vi "SO55 Ion Source Main.vi"() -> ()   [LabVIEW 2012]
panel:
  out "AnodeCurrentInd":dbl format="%#.3g"
  out "Anode Current":dbl(knob) scale=0.0..10.0
  out "GasInd":dbl format="%#.3g"
  out "Gasmeter":dbl(knob) scale=0.0..40.0
  in  "Gas":dbl(knob) min=0.0 max=40.0 step=0.1 scale=0.0..40.0
  in  "ExitBtn":bool
  in  "SetBtn":bool
  out "AnodeInd":dbl format="%#.3g"
  out "Anodemeter":dbl(knob) scale=0.0..250.0 scale format="%-#3.3p"
  in  "Anode":dbl(knob) min=0.0 max=250.0 step=1.0 scale=0.0..250.0
  out "OvenInd":dbl format="%#.3g"
  out "MagInd":dbl format="%#.3g"
  out "FilInd":dbl format="%#.3g"
  out "Ovenmeter":dbl(knob) scale=0.0..40.0
  out "Magmeter":dbl(knob) scale=0.0..40.0
  out "Filmeter":dbl(knob) scale=0.0..40.0 scale format="%-#3.3p"
  in  "Oven":dbl(knob) min=0.0 max=40.0 step=0.1 scale=0.0..40.0
  in  "Mag":dbl(knob) min=0.0 max=30.0 step=0.1 scale=0.0..40.0
  in  "Fil":dbl(knob) min=0.0 max=40.0 step=0.1 scale=0.0..40.0
  # "Magnet"
  # "Oven"
  # "Gas"
  # "Anode"
  # "Filament"
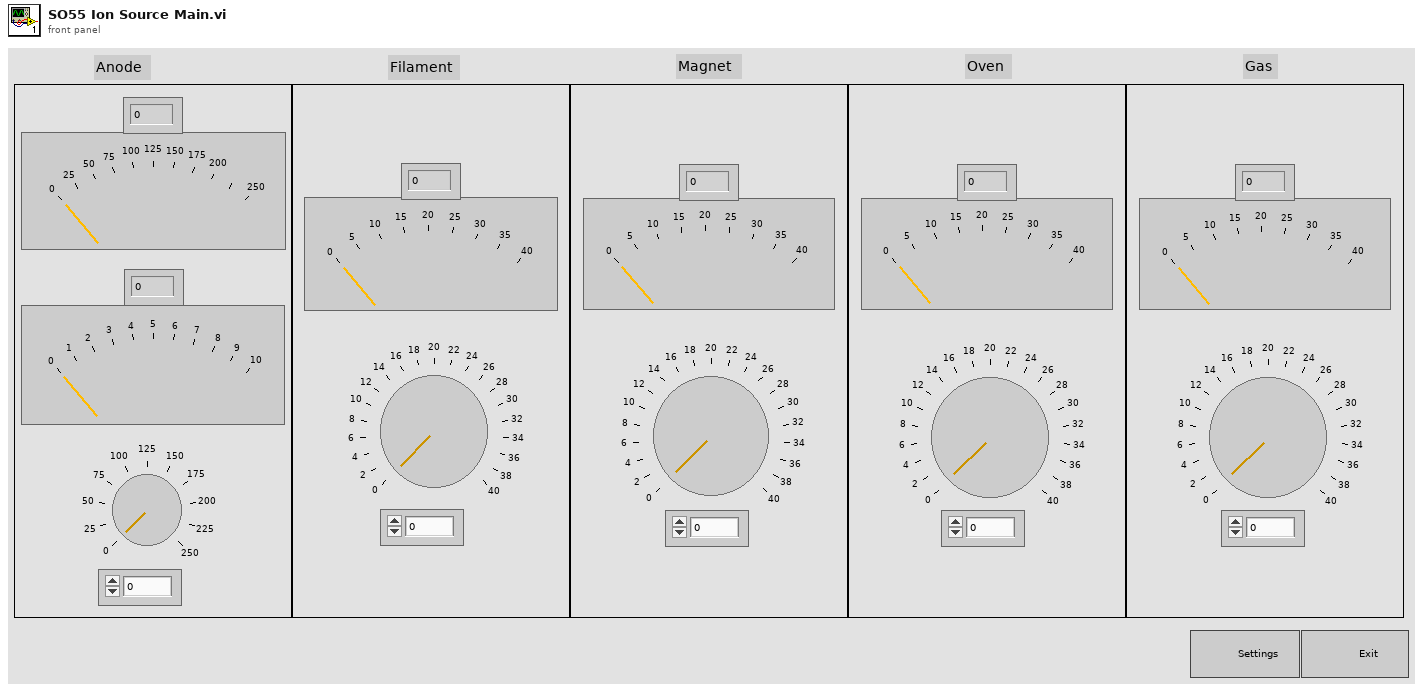
[diagram p1: front panel]
types:
  T1 = cluster{"Input":cluster{"Anode Input Channel":tag, "Filament Input Channel":tag, "Magnet Input Channel":tag, "Oven Input Channel":tag, "Gas Input Channel":tag, "Input Rate":dbl, "Anode Current Input Channel":tag}, "Output":cluster{"Anode":cluster{"Anode Output Channel":tag, "Anode Step":dbl}, "Filament":cluster{"Filament Output Channel":tag, "Filament Step":dbl}, "Magnet":cluster{"Magnet Output Channel":tag, "Magnet Step":dbl}, "Oven":cluster{"Oven Output Channel":tag, "Oven Step":dbl}, "Gas":cluster{"Gas Output Channel":tag, "Gas Step":dbl}, "Output Rate":dbl}}
  T2 = cluster{"Anode":cluster{"Anode Output Channel":tag, "Anode Step":dbl}, "Filament":cluster{"Filament Output Channel":tag, "Filament Step":dbl}, "Magnet":cluster{"Magnet Output Channel":tag, "Magnet Step":dbl}, "Oven":cluster{"Oven Output Channel":tag, "Oven Step":dbl}, "Gas":cluster{"Gas Output Channel":tag, "Gas Step":dbl}, "Output Rate":dbl}
  T3 = cluster{"Anode Input Channel":tag, "Filament Input Channel":tag, "Magnet Input Channel":tag, "Oven Input Channel":tag, "Gas Input Channel":tag, "Input Rate":dbl, "Anode Current Input Channel":tag}
  T4 = enum8{"Enabled", "Disabled", "Disabled and Grayed Out"}
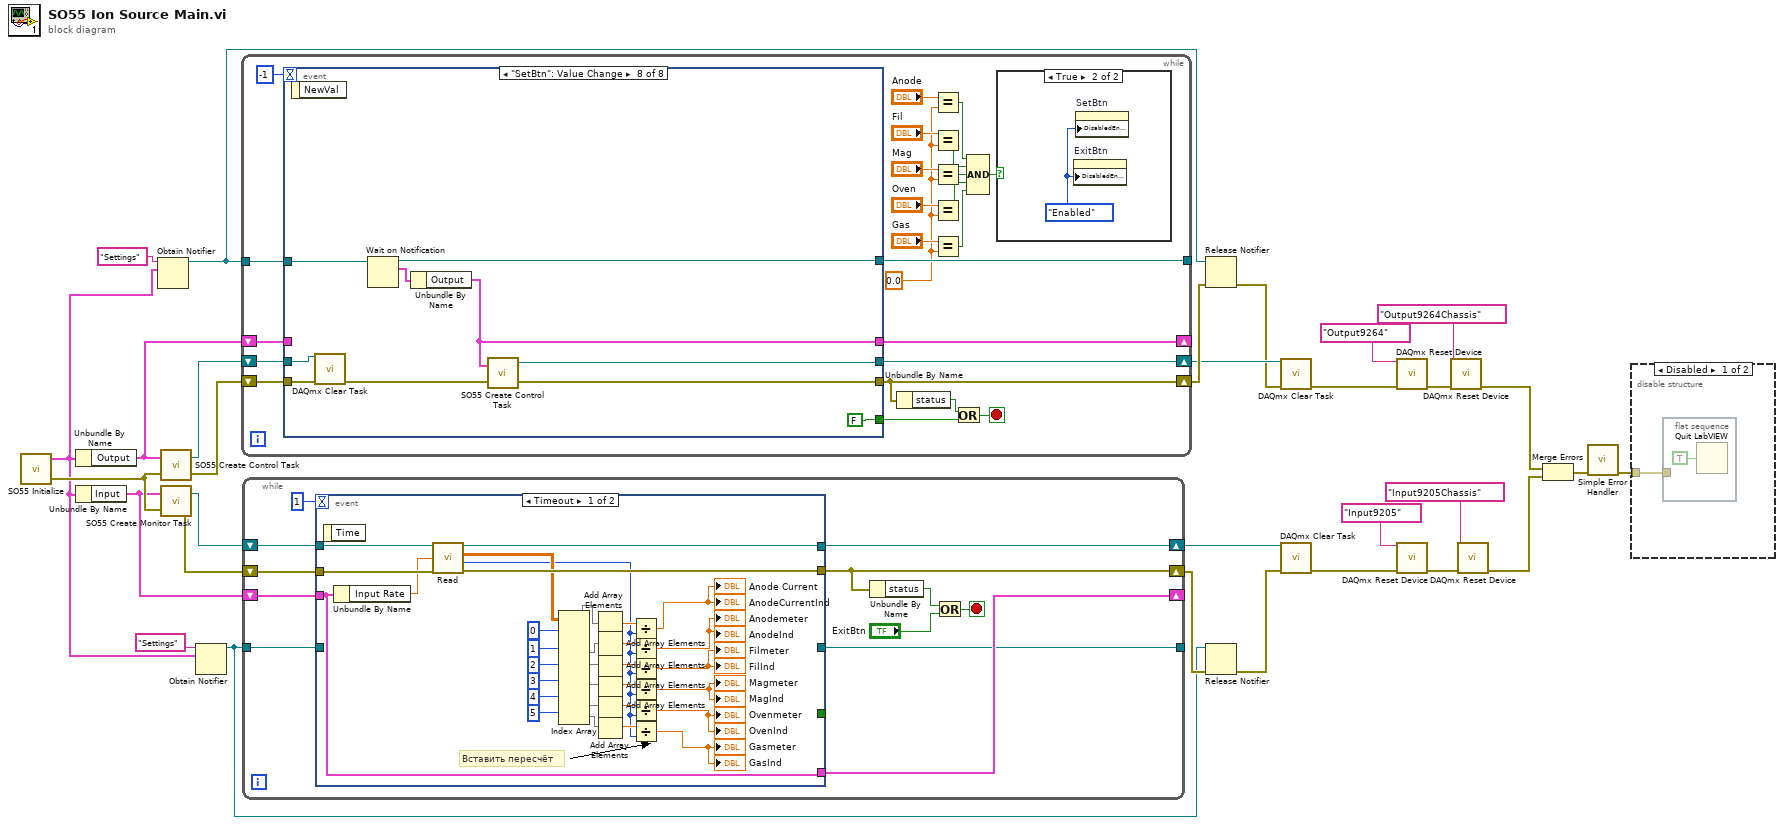
[diagram p0: block diagram]
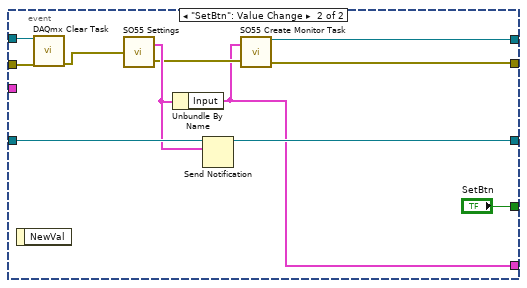
[diagram p3: hidden frame]
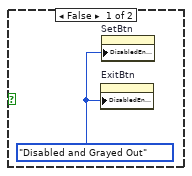
[diagram p4: hidden frame]
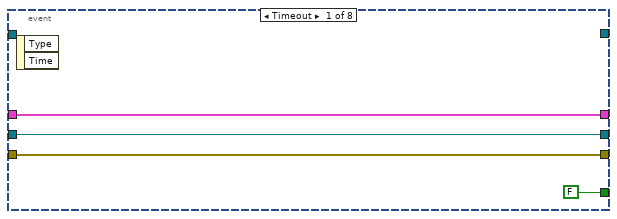
[diagram p5: hidden frame]
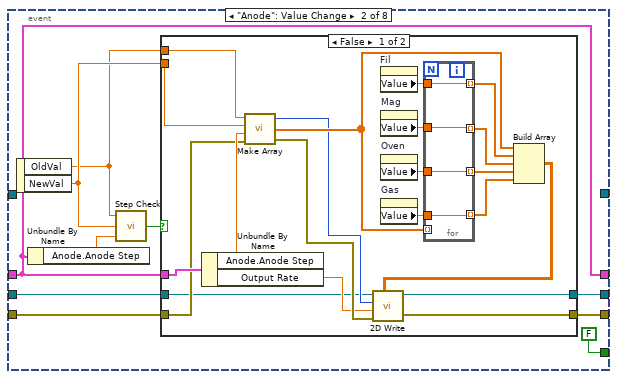
[diagram p6: hidden frame]
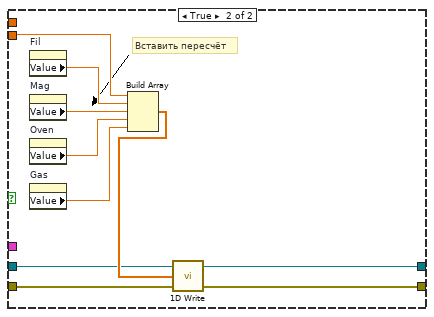
[diagram p7: hidden frame]
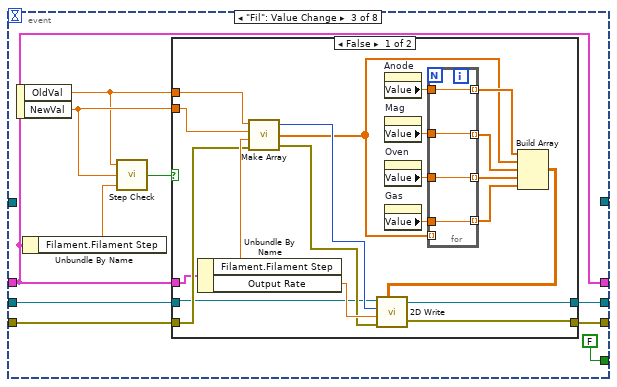
[diagram p8: hidden frame]
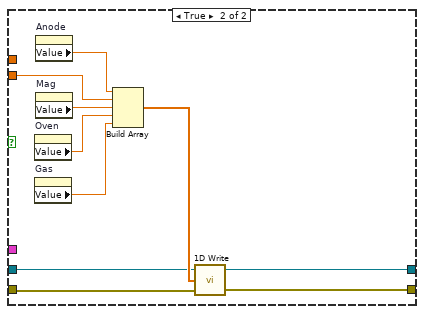
[diagram p9: hidden frame]
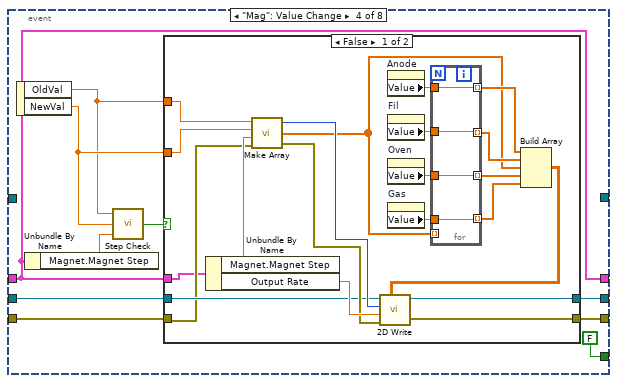
[diagram p10: hidden frame]
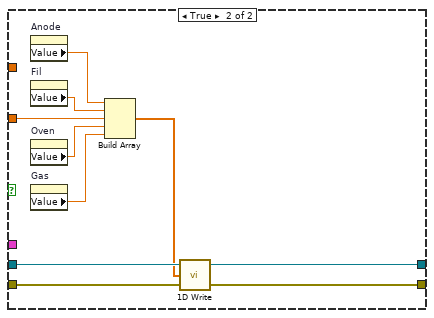
[diagram p11: hidden frame]
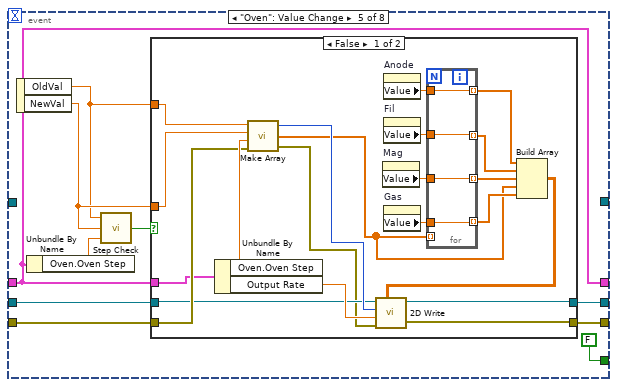
[diagram p12: hidden frame]
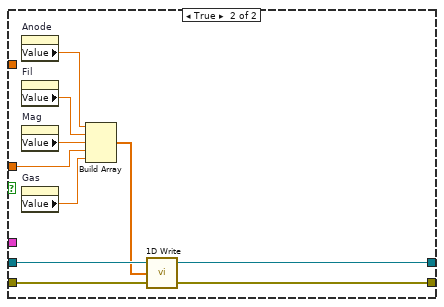
[diagram p13: hidden frame]
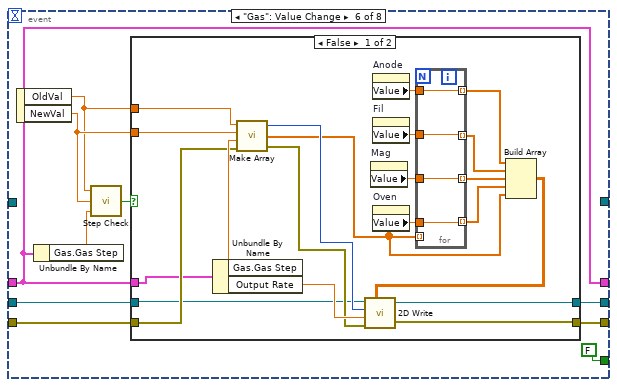
[diagram p14: hidden frame]
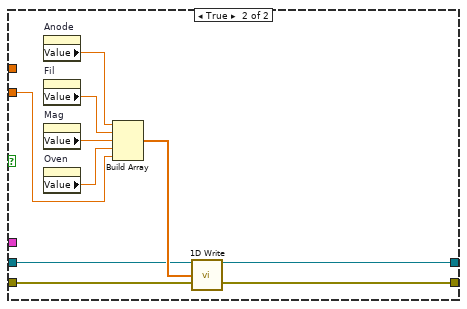
[diagram p15: hidden frame]
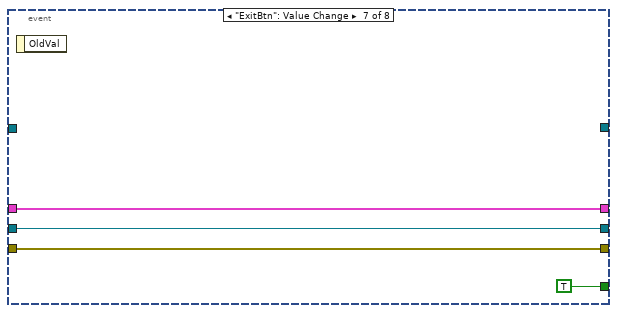
[diagram p16: hidden frame]
diagram:
  n1 = call "SO55 Initialize.vi"() -> ("error out"=w30:errorcluster, "Settings Out"=w21:T1)  [unwired: 1 in]
  n2 = Unbundle By Name(w21) -> ("Output"=w24:T2)
  n3 = Unbundle By Name(w21) -> ("Input"=w25:T3)
  n4 = Obtain Notifier(name (unnamed)="Settings", notification data type=w21) -> (notifier out=w1:refnum<notifier>)  [unwired: 2 in, 2 out]
  n5 = call "SO55 Create Control Task.vi"("error in"=w30, "Output"=w24) -> ("error out"=w26:errorcluster, "task out"=w27:refnum<k21>)
  n6 = call "SO55 Create Monitor Task.vi"("error in"=w30, "Input"=w25) -> ("error out"=w28:errorcluster, "task out"=w29:refnum<k21>)
  n7 = Obtain Notifier(name (unnamed)="Settings", notification data type=w21) -> (notifier out=w2:refnum<notifier>)  [unwired: 2 in, 2 out]
  n8 = while {
    shift-right: [w48] -> w20
    shift-left: w26 -> [w51]
    shift-right: [w53] -> w18
    shift-left: w27 -> [w52]
    shift-right: [w49] -> _
    shift-left: w24 -> [w50]
    tunnel: w1 -> [w44]
    tunnel: [w43] -> _
    stop <- w45 stop-if-true
    w37 = 0.0
    n9 = event shown="[7] \"SetBtn\": Value Change" {
      selector: _ -> [_ _ _ _ _ _ _ _]
      dyn-events: _ -> [_ _ _ _ _ _ _ _]
      timeout: -1 -> [_ _ _ _ _ _ _ _]
      tunnel: [w60 w68 w113 w155 w200 w245 w287 w292] -> w53
      tunnel: w52 -> [w60 w70 w115 w157 w202 w247 w287 w297]
      tunnel: [w59 w67 w112 w154 w199 w244 w286 w291] -> w48
      tunnel: w51 -> [w59 w69 w114 w156 w201 w246 w286 w298]
      tunnel: [w58 w61 w106 w151 w196 w241 w288 w290] -> w49
      tunnel: w50 -> [w58 w61 w106 w151 w196 w241 w288 _]
      tunnel: [FALSE FALSE FALSE FALSE FALSE FALSE TRUE FALSE] -> w46
      tunnel: w44 -> [_ _ _ _ _ _ _ w296]
      tunnel: [_ _ _ _ _ _ _ w295] -> w43
      event Timeout {
        n10 = event-data() -> ()  [unwired: 1 in, 2 out]
      }
      event "Anode": Value Change {
        n11 = event-data() -> ("OldVal"=w62:dbl, "NewVal"=w65:dbl)  [unwired: 1 in]
        n12 = Unbundle By Name(w61) -> ("Anode.Anode Step"=w64:dbl)
        n13 = call "Step Check.vi"("Step"=w64, "New Value"=w65, "Old Value"=w62) -> ("Instant output"=w66:bool)
        n14 = case shown="False" w66 {
          tunnel: w65 -> [w89 w105]
          tunnel: w70 -> [w71 w99]
          tunnel: w69 -> [w87 w98]
          tunnel: [w73 w97] -> w68
          tunnel: [w72 w96] -> w67
          tunnel: w62 -> [w90 _]
          tunnel: w61 -> [w91 _]
          frame False {
            n15 = Unbundle By Name(w91) -> ("Anode.Anode Step"=w88:dbl, "Output Rate"=w74:dbl)
            n16 = call "Make Array.vi"("Error In"=w87, "Step"=w88, "New"=w89, "Old"=w90) -> ("Error Out"=w76:errorcluster, "Array"=w78:dbl[], "Samples"=w75:i32)
            n17 = property on="Fil" class="Knob (strict)"() -> ("Value"=w86:dbl)  [unwired: 2 in, 2 out]
            n18 = property on="Mag" class="Knob (strict)"() -> ("Value"=w85:dbl)  [unwired: 2 in, 2 out]
            n19 = property on="Oven" class="Knob (strict)"() -> ("Value"=w84:dbl)  [unwired: 2 in, 2 out]
            n20 = property on="Gas" class="Knob (strict)"() -> ("Value"=w83:dbl)  [unwired: 2 in, 2 out]
            n21 = for {
              tunnel: w86 -> [w95]
              tunnel: w85 -> [w94]
              tunnel: w78 -> [_] mode=indexing
              tunnel: w84 -> [w93]
              tunnel: w83 -> [w92]
              tunnel: [w95] -> w79 mode=indexing
              tunnel: [w94] -> w80 mode=indexing
              tunnel: [w93] -> w81 mode=indexing
              tunnel: [w92] -> w82 mode=indexing
            }
            n22 = Build Array(w78, w79, w80, w81, w82) -> (w77:dbl[][])
            n23 = call "2D Write.vi"("Task"=w71, "samples per channel"=w75, "rate"=w74, "Error In"=w76, "data"=w77) -> ("task out"=w73:refnum<k21>, "Error Out"=w72:errorcluster)
          }
          frame True {
            # "Вставить пересчёт"
            n24 = property on="Fil" class="Knob (strict)"() -> ("Value"=w101:dbl)  [unwired: 2 in, 2 out]
            n25 = property on="Mag" class="Knob (strict)"() -> ("Value"=w104:dbl)  [unwired: 2 in, 2 out]
            n26 = property on="Oven" class="Knob (strict)"() -> ("Value"=w103:dbl)  [unwired: 2 in, 2 out]
            n27 = property on="Gas" class="Knob (strict)"() -> ("Value"=w102:dbl)  [unwired: 2 in, 2 out]
            n28 = Build Array(w105, w101, w104, w103, w102) -> (w100:dbl[])
            n29 = call "1D Write.vi"("error in (no error)"=w98, "Data Array"=w100, "Task in"=w99) -> ("error out"=w96:errorcluster, "Task out"=w97:refnum<k21>)
          }
        }
      }
      event "Fil": Value Change {
        n30 = event-data() -> ("OldVal"=w107:dbl, "NewVal"=w109:dbl)  [unwired: 1 in]
        n31 = Unbundle By Name(w106) -> ("Filament.Filament Step"=w110:dbl)
        n32 = call "Step Check.vi"("Step"=w110, "New Value"=w109, "Old Value"=w107) -> ("Instant output"=w111:bool)
        n33 = case shown="False" w111 {
          tunnel: w109 -> [w117 w149]
          tunnel: w115 -> [w120 w144]
          tunnel: w114 -> [w123 w143]
          tunnel: [w119 w142] -> w113
          tunnel: [w121 w141] -> w112
          tunnel: w106 -> [w118 _]
          tunnel: w107 -> [w116 _]
          frame False {
            n34 = Unbundle By Name(w118) -> ("Filament.Filament Step"=w136:dbl, "Output Rate"=w127:dbl)
            n35 = call "Make Array.vi"("Error In"=w123, "Step"=w136, "New"=w117, "Old"=w116) -> ("Error Out"=w122:errorcluster, "Array"=w124:dbl[], "Samples"=w128:i32)
            n36 = property on="Anode" class="Knob (strict)"() -> ("Value"=w126:dbl)  [unwired: 2 in, 2 out]
            n37 = property on="Mag" class="Knob (strict)"() -> ("Value"=w135:dbl)  [unwired: 2 in, 2 out]
            n38 = property on="Oven" class="Knob (strict)"() -> ("Value"=w134:dbl)  [unwired: 2 in, 2 out]
            n39 = property on="Gas" class="Knob (strict)"() -> ("Value"=w133:dbl)  [unwired: 2 in, 2 out]
            n40 = for {
              tunnel: w126 -> [w140]
              tunnel: w135 -> [w139]
              tunnel: w124 -> [_] mode=indexing
              tunnel: w134 -> [w138]
              tunnel: w133 -> [w137]
              tunnel: [w140] -> w125 mode=indexing
              tunnel: [w139] -> w130 mode=indexing
              tunnel: [w138] -> w131 mode=indexing
              tunnel: [w137] -> w132 mode=indexing
            }
            n41 = Build Array(w125, w124, w130, w131, w132) -> (w129:dbl[][])
            n42 = call "2D Write.vi"("Task"=w120, "samples per channel"=w128, "rate"=w127, "Error In"=w122, "data"=w129) -> ("task out"=w119:refnum<k21>, "Error Out"=w121:errorcluster)
          }
          frame True {
            n43 = property on="Oven" class="Knob (strict)"() -> ("Value"=w147:dbl)  [unwired: 2 in, 2 out]
            n44 = property on="Gas" class="Knob (strict)"() -> ("Value"=w146:dbl)  [unwired: 2 in, 2 out]
            n45 = property on="Anode" class="Knob (strict)"() -> ("Value"=w150:dbl)  [unwired: 2 in, 2 out]
            n46 = property on="Mag" class="Knob (strict)"() -> ("Value"=w148:dbl)  [unwired: 2 in, 2 out]
            n47 = Build Array(w150, w149, w148, w147, w146) -> (w145:dbl[])
            n48 = call "1D Write.vi"("error in (no error)"=w143, "Data Array"=w145, "Task in"=w144) -> ("error out"=w141:errorcluster, "Task out"=w142:refnum<k21>)
          }
        }
      }
      event "Mag": Value Change {
        n49 = event-data() -> ("OldVal"=w152:dbl, "NewVal"=w158:dbl)  [unwired: 1 in]
        n50 = Unbundle By Name(w151) -> ("Magnet.Magnet Step"=w159:dbl)
        n51 = call "Step Check.vi"("Step"=w159, "New Value"=w158, "Old Value"=w152) -> ("Instant output"=w160:bool)
        n52 = case shown="False" w160 {
          tunnel: w158 -> [w166 w191]
          tunnel: w157 -> [w168 w195]
          tunnel: w156 -> [w167 w194]
          tunnel: [w170 w193] -> w155
          tunnel: [w169 w192] -> w154
          tunnel: w152 -> [w165 _]
          tunnel: w151 -> [w161 _]
          frame False {
            n53 = Unbundle By Name(w161) -> ("Magnet.Magnet Step"=w181:dbl, "Output Rate"=w174:dbl)
            n54 = call "Make Array.vi"("Error In"=w167, "Step"=w181, "New"=w166, "Old"=w165) -> ("Error Out"=w171:errorcluster, "Array"=w162:dbl[], "Samples"=w175:i32)
            n55 = property on="Anode" class="Knob (strict)"() -> ("Value"=w173:dbl)  [unwired: 2 in, 2 out]
            n56 = property on="Fil" class="Knob (strict)"() -> ("Value"=w164:dbl)  [unwired: 2 in, 2 out]
            n57 = property on="Oven" class="Knob (strict)"() -> ("Value"=w180:dbl)  [unwired: 2 in, 2 out]
            n58 = property on="Gas" class="Knob (strict)"() -> ("Value"=w179:dbl)  [unwired: 2 in, 2 out]
            n59 = for {
              tunnel: w173 -> [w185]
              tunnel: w164 -> [w184]
              tunnel: w162 -> [_] mode=indexing
              tunnel: w180 -> [w183]
              tunnel: w179 -> [w182]
              tunnel: [w185] -> w172 mode=indexing
              tunnel: [w184] -> w163 mode=indexing
              tunnel: [w183] -> w177 mode=indexing
              tunnel: [w182] -> w178 mode=indexing
            }
            n60 = Build Array(w172, w163, w162, w177, w178) -> (w176:dbl[][])
            n61 = call "2D Write.vi"("Task"=w168, "samples per channel"=w175, "rate"=w174, "Error In"=w171, "data"=w176) -> ("task out"=w170:refnum<k21>, "Error Out"=w169:errorcluster)
          }
          frame True {
            n62 = property on="Anode" class="Knob (strict)"() -> ("Value"=w189:dbl)  [unwired: 2 in, 2 out]
            n63 = property on="Fil" class="Knob (strict)"() -> ("Value"=w190:dbl)  [unwired: 2 in, 2 out]
            n64 = property on="Oven" class="Knob (strict)"() -> ("Value"=w188:dbl)  [unwired: 2 in, 2 out]
            n65 = property on="Gas" class="Knob (strict)"() -> ("Value"=w187:dbl)  [unwired: 2 in, 2 out]
            n66 = Build Array(w189, w190, w191, w188, w187) -> (w186:dbl[])
            n67 = call "1D Write.vi"("error in (no error)"=w194, "Data Array"=w186, "Task in"=w195) -> ("error out"=w192:errorcluster, "Task out"=w193:refnum<k21>)
          }
        }
      }
      event "Oven": Value Change {
        n68 = event-data() -> ("OldVal"=w197:dbl, "NewVal"=w203:dbl)  [unwired: 1 in]
        n69 = Unbundle By Name(w196) -> ("Oven.Oven Step"=w204:dbl)
        n70 = call "Step Check.vi"("Step"=w204, "New Value"=w203, "Old Value"=w197) -> ("Instant output"=w205:bool)
        n71 = case shown="False" w205 {
          tunnel: w203 -> [w212 w239]
          tunnel: w202 -> [w213 w235]
          tunnel: w201 -> [w214 w234]
          tunnel: [w216 w233] -> w200
          tunnel: [w215 w232] -> w199
          tunnel: w197 -> [w211 _]
          tunnel: w196 -> [w210 _]
          frame False {
            n72 = Unbundle By Name(w210) -> ("Oven.Oven Step"=w226:dbl, "Output Rate"=w221:dbl)
            n73 = call "Make Array.vi"("Error In"=w214, "Step"=w226, "New"=w212, "Old"=w211) -> ("Error Out"=w209:errorcluster, "Array"=w206:dbl[], "Samples"=w222:i32)
            n74 = property on="Mag" class="Knob (strict)"() -> ("Value"=w207:dbl)  [unwired: 2 in, 2 out]
            n75 = property on="Anode" class="Knob (strict)"() -> ("Value"=w220:dbl)  [unwired: 2 in, 2 out]
            n76 = property on="Fil" class="Knob (strict)"() -> ("Value"=w218:dbl)  [unwired: 2 in, 2 out]
            n77 = property on="Gas" class="Knob (strict)"() -> ("Value"=w225:dbl)  [unwired: 2 in, 2 out]
            n78 = for {
              tunnel: w220 -> [w230]
              tunnel: w218 -> [w229]
              tunnel: w206 -> [_] mode=indexing
              tunnel: w207 -> [w228]
              tunnel: w225 -> [w227]
              tunnel: [w230] -> w219 mode=indexing
              tunnel: [w229] -> w217 mode=indexing
              tunnel: [w228] -> w208 mode=indexing
              tunnel: [w227] -> w224 mode=indexing
            }
            n79 = Build Array(w219, w217, w208, w206, w224) -> (w223:dbl[][])
            n80 = call "2D Write.vi"("Task"=w213, "samples per channel"=w222, "rate"=w221, "Error In"=w209, "data"=w223) -> ("task out"=w216:refnum<k21>, "Error Out"=w215:errorcluster)
          }
          frame True {
            n81 = property on="Anode" class="Knob (strict)"() -> ("Value"=w236:dbl)  [unwired: 2 in, 2 out]
            n82 = property on="Fil" class="Knob (strict)"() -> ("Value"=w237:dbl)  [unwired: 2 in, 2 out]
            n83 = property on="Mag" class="Knob (strict)"() -> ("Value"=w238:dbl)  [unwired: 2 in, 2 out]
            n84 = property on="Gas" class="Knob (strict)"() -> ("Value"=w240:dbl)  [unwired: 2 in, 2 out]
            n85 = Build Array(w236, w237, w238, w239, w240) -> (w231:dbl[])
            n86 = call "1D Write.vi"("error in (no error)"=w234, "Data Array"=w231, "Task in"=w235) -> ("error out"=w232:errorcluster, "Task out"=w233:refnum<k21>)
          }
        }
      }
      event "Gas": Value Change {
        n87 = event-data() -> ("OldVal"=w242:dbl, "NewVal"=w248:dbl)  [unwired: 1 in]
        n88 = Unbundle By Name(w241) -> ("Gas.Gas Step"=w249:dbl)
        n89 = call "Step Check.vi"("Step"=w249, "New Value"=w248, "Old Value"=w242) -> ("Instant output"=w250:bool)
        n90 = case shown="False" w250 {
          tunnel: w248 -> [w256 w281]
          tunnel: w247 -> [w259 w279]
          tunnel: w246 -> [w260 w278]
          tunnel: [w262 w277] -> w245
          tunnel: [w261 w276] -> w244
          tunnel: w241 -> [w258 _]
          tunnel: w242 -> [w257 _]
          frame False {
            n91 = Unbundle By Name(w258) -> ("Gas.Gas Step"=w271:dbl, "Output Rate"=w268:dbl)
            n92 = call "Make Array.vi"("Error In"=w260, "Step"=w271, "New"=w256, "Old"=w257) -> ("Error Out"=w265:errorcluster, "Array"=w251:dbl[], "Samples"=w269:i32)
            n93 = property on="Mag" class="Knob (strict)"() -> ("Value"=w254:dbl)  [unwired: 2 in, 2 out]
            n94 = property on="Anode" class="Knob (strict)"() -> ("Value"=w267:dbl)  [unwired: 2 in, 2 out]
            n95 = property on="Fil" class="Knob (strict)"() -> ("Value"=w264:dbl)  [unwired: 2 in, 2 out]
            n96 = property on="Oven" class="Knob (strict)"() -> ("Value"=w255:dbl)  [unwired: 2 in, 2 out]
            n97 = for {
              tunnel: w267 -> [w275]
              tunnel: w264 -> [w274]
              tunnel: w251 -> [_] mode=indexing
              tunnel: w254 -> [w273]
              tunnel: w255 -> [w272]
              tunnel: [w275] -> w266 mode=indexing
              tunnel: [w274] -> w263 mode=indexing
              tunnel: [w273] -> w253 mode=indexing
              tunnel: [w272] -> w252 mode=indexing
            }
            n98 = Build Array(w266, w263, w253, w252, w251) -> (w270:dbl[][])
            n99 = call "2D Write.vi"("Task"=w259, "samples per channel"=w269, "rate"=w268, "Error In"=w265, "data"=w270) -> ("task out"=w262:refnum<k21>, "Error Out"=w261:errorcluster)
          }
          frame True {
            n100 = property on="Anode" class="Knob (strict)"() -> ("Value"=w284:dbl)  [unwired: 2 in, 2 out]
            n101 = property on="Fil" class="Knob (strict)"() -> ("Value"=w285:dbl)  [unwired: 2 in, 2 out]
            n102 = property on="Mag" class="Knob (strict)"() -> ("Value"=w283:dbl)  [unwired: 2 in, 2 out]
            n103 = property on="Oven" class="Knob (strict)"() -> ("Value"=w282:dbl)  [unwired: 2 in, 2 out]
            n104 = Build Array(w284, w285, w283, w282, w281) -> (w280:dbl[])
            n105 = call "1D Write.vi"("error in (no error)"=w278, "Data Array"=w280, "Task in"=w279) -> ("error out"=w276:errorcluster, "Task out"=w277:refnum<k21>)
          }
        }
      }
      event "ExitBtn": Value Change {
        n106 = event-data() -> ()  [unwired: 1 in, 1 out]
      }
      event "SetBtn": Value Change {
        n107 = event-data() -> ()  [unwired: 1 in, 1 out]
        n108 = call <vilib>:"DAQmx Clear Task.vi"("task in"=w297, "error in"=w298) -> ("error out"=w293:errorcluster)  [unwired: 13 in]
        n109 = Wait on Notification(notifier=w296) -> (notifier out=w295:refnum<notifier>, notification=w294:T1)  [unwired: 3 in, 2 out]
        n110 = Unbundle By Name(w294) -> ("Output"=w290:T2)
        n111 = call "SO55 Create Control Task.vi"("error in"=w293, "Output"=w290) -> ("error out"=w291:errorcluster, "task out"=w292:refnum<k21>)
      }
    }
    n112 = Unbundle By Name(w48) -> ("status"=w47:bool)
    n113 = Equal?(x="Anode", y=w37) -> (x = y?=w36:bool)
    n114 = Equal?(x="Fil", y=w37) -> (x = y?=w35:bool)
    n115 = Equal?(x="Mag", y=w37) -> (x = y?=w34:bool)
    n116 = Equal?(x="Oven", y=w37) -> (x = y?=w33:bool)
    n117 = Equal?(x="Gas", y=w37) -> (x = y?=w32:bool)
    n118 = Or(x=w47, y=w46) -> (x .or. y?=w45:bool)
    n119 = Compound Arithmetic op=AND(w36, w35, w34, w33, w32) -> (w31:bool)
    n120 = case shown="True" w31 {
      frame False {
        w55 = T4."Disabled and Grayed Out" ("Disabled")
        n121 = property on="ExitBtn" class="Bool"("DisabledEnum"=w55) -> ()  [unwired: 2 in, 2 out]
        n122 = property on="SetBtn" class="Bool"("DisabledEnum"=w55) -> ()  [unwired: 2 in, 2 out]
      }
      frame True {
        w56 = T4."Enabled" ("Disabled")
        n123 = property on="ExitBtn" class="Bool"("DisabledEnum"=w56) -> ()  [unwired: 2 in, 2 out]
        n124 = property on="SetBtn" class="Bool"("DisabledEnum"=w56) -> ()  [unwired: 2 in, 2 out]
      }
    }
  }
  n125 = while {
    shift-right: [w305] -> w19
    shift-left: w28 -> [w309]
    shift-right: [w307] -> w16
    shift-left: w29 -> [w310]
    shift-right: [w306] -> _
    shift-left: w25 -> [w308]
    tunnel: w2 -> [w301]
    tunnel: [w300] -> _
    stop <- w302 stop-if-true
    n126 = event shown="[0] Timeout" {
      selector: _ -> [_ _]
      dyn-events: _ -> [_ _]
      timeout: 1 -> [_ _]
      tunnel: [_ "SetBtn"] -> _
      tunnel: w310 -> [w343 w353]
      tunnel: w309 -> [w342 w352]
      tunnel: w308 -> [w318 _]
      tunnel: [w340 w346] -> w307
      tunnel: [w339 w345] -> w305
      tunnel: [w318 w344] -> w306
      tunnel: w301 -> [_ w350]
      tunnel: [_ w349] -> w300
      event Timeout {
        # "Вставить пересчёт"
        n127 = event-data() -> ()  [unwired: 1 in, 1 out]
        n128 = Unbundle By Name(w318) -> ("Input Rate"=w341:dbl)
        n129 = call "Read.vi"("Task in"=w343, "Input Rate"=w341, "error in (no error)"=w342) -> ("Task out"=w340:refnum<k21>, "data"=w326:dbl[][], "samples"=w314:i32, "error out"=w339:errorcluster)
        n130 = Index Array(array=w326, index (row) #1=0 ("index (row)"), index (row) #2=1 ("index (row)"), index (row) #3=2 ("index (row)"), index (row) #4=3 ("index (row)"), index (row) #5=4 ("index (row)"), index (row) #6=5 ("index (row)")) -> (element #1=w316:dbl[], element #2=w334:dbl[], element #3=w333:dbl[], element #4=w332:dbl[], element #5=w331:dbl[], element #6=w324:dbl[])  [unwired: 6 in]
        n131 = Add Array Elements(numeric array=w316) -> (sum=w315:dbl)
        n132 = Add Array Elements(numeric array=w334) -> (sum=w330:dbl)
        n133 = Add Array Elements(numeric array=w333) -> (sum=w329:dbl)
        n134 = Add Array Elements(numeric array=w332) -> (sum=w328:dbl)
        n135 = Add Array Elements(numeric array=w331) -> (sum=w327:dbl)
        n136 = Add Array Elements(numeric array=w324) -> (sum=w323:dbl)
        n137 = Divide(x=w315, y=w314) -> (x/y=→"Anode Current" →"AnodeCurrentInd":dbl)
        n138 = Divide(x=w330, y=w314) -> (x/y=→"Anodemeter" →"AnodeInd":dbl)
        n139 = Divide(x=w329, y=w314) -> (x/y=→"Filmeter" →"FilInd":dbl)
        n140 = Divide(x=w328, y=w314) -> (x/y=→"Magmeter" →"MagInd":dbl)
        n141 = Divide(x=w327, y=w314) -> (x/y=→"Ovenmeter" →"OvenInd":dbl)
        n142 = Divide(x=w323, y=w314) -> (x/y=→"Gasmeter" →"GasInd":dbl)
      }
      event "SetBtn": Value Change {
        n143 = event-data() -> ()  [unwired: 1 in, 1 out]
        n144 = call <vilib>:"DAQmx Clear Task.vi"("task in"=w353, "error in"=w352) -> ("error out"=w351:errorcluster)  [unwired: 13 in]
        n145 = call "SO55 Settings.vi"("Error In"=w351) -> ("Settings Out"=w348:T1, "Error Out"=w347:errorcluster)
        n146 = Unbundle By Name(w348) -> ("Input"=w344:T3)
        n147 = Send Notification(notification=w348, notifier=w350) -> (notifier out=w349:refnum<notifier>)  [unwired: 1 in, 1 out]
        n148 = call "SO55 Create Monitor Task.vi"("error in"=w347, "Input"=w344) -> ("error out"=w345:errorcluster, "task out"=w346:refnum<k21>)
      }
    }
    n149 = Unbundle By Name(w305) -> ("status"=w304:bool)
    n150 = Or(x=w304, y="ExitBtn") -> (x .or. y?=w302:bool)
  }
  n151 = Release Notifier(notifier=w1, error in (no error)=w20) -> (error out=w17:errorcluster)  [unwired: 1 in, 2 out]
  n152 = Release Notifier(notifier=w2, error in (no error)=w19) -> (error out=w15:errorcluster)  [unwired: 1 in, 2 out]
  n153 = call <vilib>:"DAQmx Clear Task.vi"("task in"=w18, "error in"=w17) -> ("error out"=w14:errorcluster)  [unwired: 13 in]
  n154 = call <vilib>:"DAQmx Clear Task.vi"("task in"=w16, "error in"=w15) -> ("error out"=w11:errorcluster)  [unwired: 13 in]
  n155 = call <vilib>:"DAQmx Reset Device.vi"("device in"=tag "Output9264", "error in"=w14) -> ("error out"=w8:errorcluster)  [unwired: 13 in]
  n156 = call <vilib>:"DAQmx Reset Device.vi"("device in"=tag "Input9205", "error in"=w11) -> ("error out"=w5:errorcluster)  [unwired: 13 in]
  n157 = call <vilib>:"DAQmx Reset Device.vi"("device in"=tag "Output9264Chassis", "error in"=w8) -> ("error out"=w7:errorcluster)  [unwired: 13 in]
  n158 = call <vilib>:"DAQmx Reset Device.vi"("device in"=tag "Input9205Chassis", "error in"=w5) -> ("error out"=w4:errorcluster)  [unwired: 13 in]
  n159 = Merge Errors(w7, w4) -> (w10:errorcluster)
  n160 = call <vilib>:"Simple Error Handler.vi"("error in (no error)"=w10) -> ("error out"=w9:errorcluster)  [unwired: 4 in, 4 out]
  n161 = disable-structure shown="Disabled" {
    disable-tunnel: w9 -> [w355 _]
    frame Disabled {
      n162 = flat-sequence {
        tunnel: w355 -> [_]
        frame #0 {
          n163 = Quit LabVIEW(quit? (T)=TRUE) -> ()
        }
      }
    }
    frame Enabled {
    }
  }
